vi "Script Controls (XML).vi"(11 "IDM Descriptor Array In":T1) -> (0 "error out":errorcluster, 1 "Terms to Show":string[](array[string]), 2 "Generated XML":string, 3 "IDM Descriptor Array Out":T1, 4 "Required Terms":i32[](array[numeric]))   [LabVIEW 2021]
uses:
  <vilib>/myRIO/Common/Express VI Framework/typedefs/Instrument Driver Method Descriptor Array.ctl
  <vilib>/myRIO/Common/Express VI Framework/typedefs/Instrument Driver Method Descriptor.ctl
  <vilib>/myRIO/Common/Express VI Framework/typedefs/Create FP Controls Actions.ctl
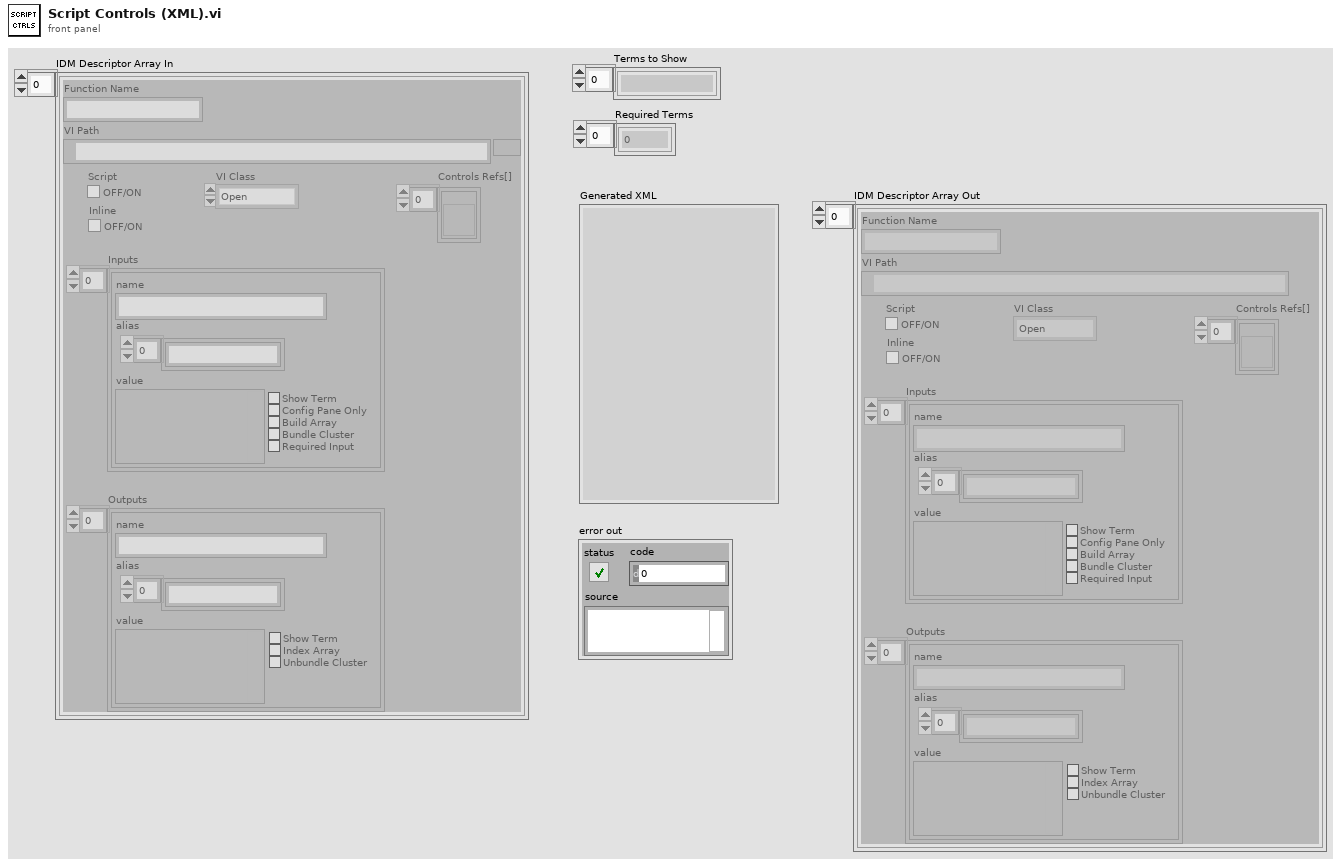
[diagram p1: front panel]
types:
  T1 = typedef "Instrument Driver Method Descriptor Array.ctl" = T2[]
  T2 = typedef "Instrument Driver Method Descriptor.ctl" = cluster{"Function Name":string, "VI Path":path, "Script":bool, "Inputs":cluster{"name":string, "value":variant, "Config Pane Only":bool, "Build Array":bool, "Bundle Cluster":bool, "Show Term":bool, "alias":string[], "Required Input":bool}[], "Outputs":cluster{"name":string, "value":variant, "Show Term":bool, "Index Array":bool, "Unbundle Cluster":bool, "alias":string[]}[], "VI Class":enum16{"Open", "Configure", "Data", "Manage", "Close"}, "Controls Refs[]":refnum<vi>[], "Inline":bool}
  T3 = typedef "Create FP Controls Actions.ctl" = enum16{"Create Control", "Create Indicator", "Create Constant", "Build Array", "Index Array", "Create Error In", "Create Error Out", "Bundle Cluster", "Unbundle Cluster"}
  T4 = cluster{"name":string, "value":variant, "Config Pane Only":bool, "Build Array":bool, "Bundle Cluster":bool, "Show Term":bool, "alias":string[], "Required Input":bool}[]
  T5 = cluster{"name":string, "value":variant, "Show Term":bool, "Index Array":bool, "Unbundle Cluster":bool, "alias":string[]}[]
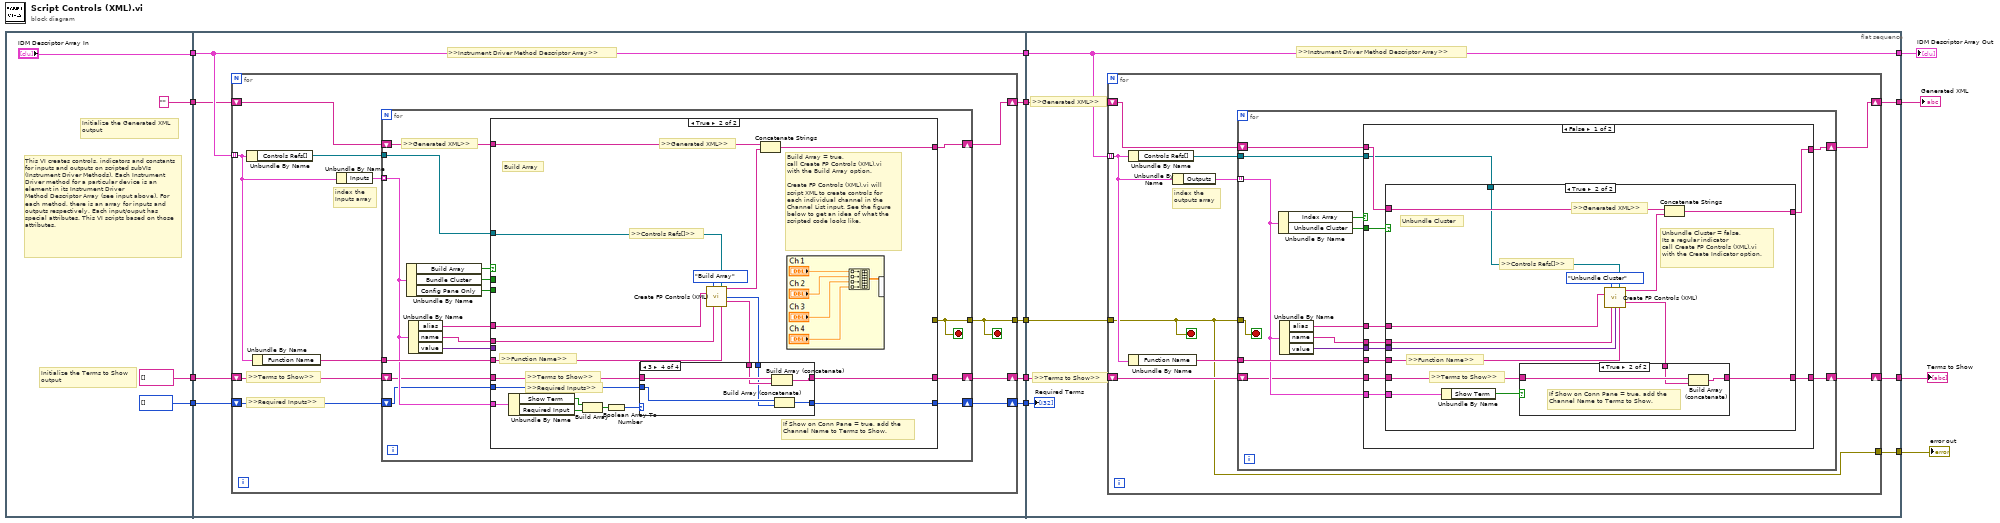
[diagram p0: block diagram]
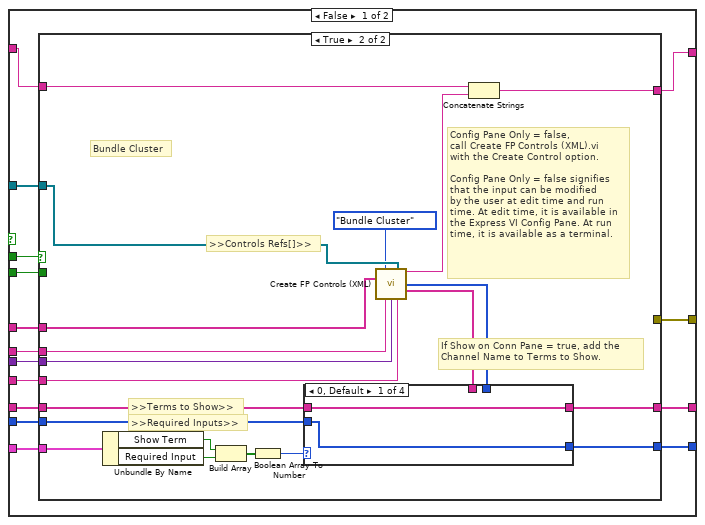
[diagram p2: hidden frame]
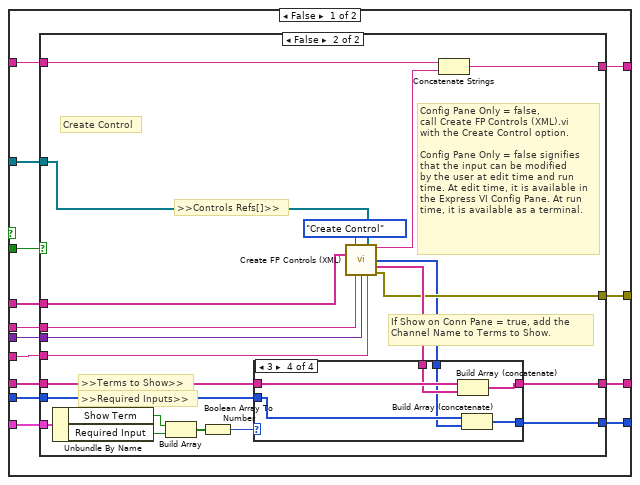
[diagram p3: hidden frame]
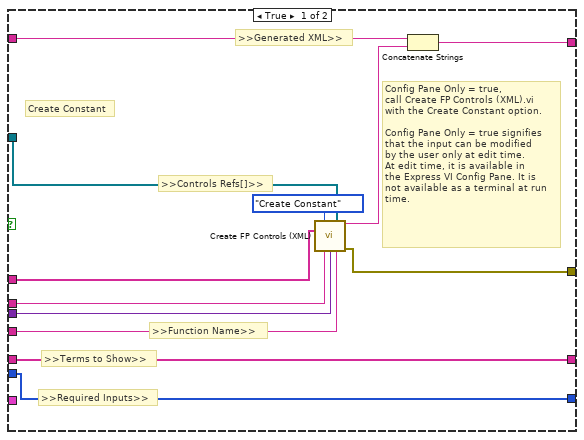
[diagram p4: hidden frame]
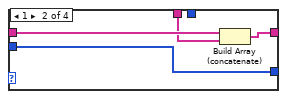
[diagram p6: hidden frame]
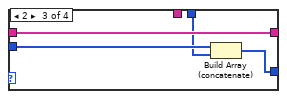
[diagram p7: hidden frame]
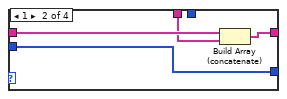
[diagram p8: hidden frame]
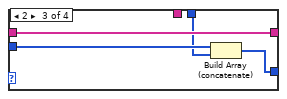
[diagram p9: hidden frame]
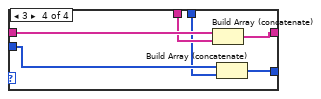
[diagram p10: hidden frame]
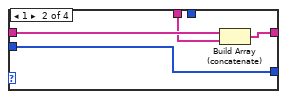
[diagram p12: hidden frame]
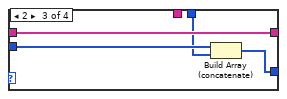
[diagram p13: hidden frame]
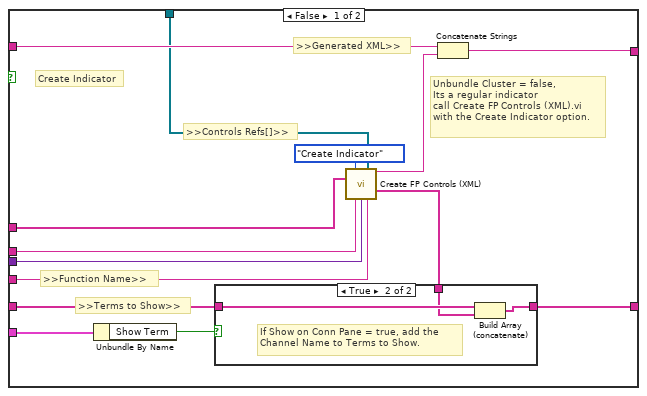
[diagram p14: hidden frame]
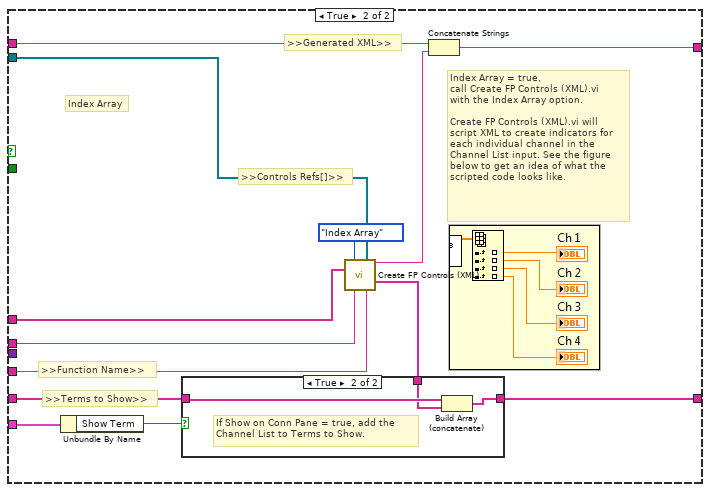
[diagram p17: hidden frame]
diagram:
  n1 = flat-sequence {
    tunnel: ["IDM Descriptor Array In"] -> w13
    tunnel: ["" ("Generated XML")] -> w11
    tunnel: [string[] [] ("array")] -> w8
    tunnel: [i32[] [] ("Required Terms")] -> w2
    tunnel: w13 -> [w25]
    tunnel: [w25] -> w12
    tunnel: w11 -> [w24]
    tunnel: [w23] -> w10
    tunnel: w8 -> [w22]
    tunnel: [w21] -> w7
    tunnel: [w20] -> w4
    tunnel: w2 -> [w19]
    tunnel: [w18] -> w1
    tunnel: w12 -> [w205]
    tunnel: w10 -> [w209]
    tunnel: [w208] -> w9
    tunnel: w7 -> [w207]
    tunnel: [w206] -> w6
    tunnel: [w205] -> w5
    tunnel: w4 -> [w204]
    tunnel: [w203] -> w3
    tunnel: w1 -> [w202]
    frame #0 {
      # "This VI creates controls, indicators and constants for inputs and outputs on scripted subVIs (Instrument Driver Methods). Each Instrument Driver method for a particular device is an element in its Instrument Driver \nMethod Descriptor Array (see input above). For each method, there is an array for inputs and outputs respectively. Each input/ouput has special attributes. This VI scripts based on those attributes."
      # "Initialize the Terms to Show\noutput"
      # "Initialize the Generated XML\noutput"
    }
    frame #1 {
      # ">>Instrument Driver Method Descriptor Array>>"
      n2 = for {
        tunnel: w25 -> [w36] mode=indexing
        shift-right: [w33] -> w23
        shift-left: w24 -> [w34]
        shift-right: [w31] -> w21
        shift-left: w22 -> [w32]
        tunnel: [w28] -> w20
        shift-right: [w26] -> w18
        shift-left: w19 -> [w27]
        stop <- w28 stop-if-true
        # ">>Required Inputs>>"
        # "index the \nInputs array"
        # ">>Terms to Show>>"
        n3 = Unbundle By Name(w36) -> ("Controls Refs[]"=w30:refnum<vi>[])
        n4 = Unbundle By Name(w36) -> ("Function Name"=w35:string)
        n5 = Unbundle By Name(w36) -> ("Inputs"=w29:T4)
        n6 = for {
          tunnel: w29 -> [w48] mode=indexing
          tunnel: w35 -> [w50]
          shift-right: [w44] -> w33
          shift-left: w34 -> [w45]
          tunnel: w30 -> [w43]
          shift-right: [w41] -> w31
          shift-left: w32 -> [w42]
          tunnel: [w39] -> w28
          shift-right: [w37] -> w26
          shift-left: w27 -> [w38]
          stop <- w39 stop-if-true
          # ">>Generated XML>>"
          n7 = Unbundle By Name(w48) -> ("Build Array"=w47:bool, "Bundle Cluster"=w46:bool, "Config Pane Only"=w52:bool)
          n8 = Unbundle By Name(w48) -> ("alias"=w40:string[], "name"=w51:string, "value"=w49:variant)
          n9 = case shown="True" w47 {
            tunnel: w52 -> [w67 _]
            tunnel: w51 -> [w66 w184]
            tunnel: w50 -> [w65 w183]
            tunnel: w49 -> [w64 _]
            tunnel: w48 -> [w63 w174]
            tunnel: w46 -> [w62 _]
            tunnel: w45 -> [w61 w181]
            tunnel: [w60 w182] -> w44
            tunnel: w43 -> [w59 w180]
            tunnel: w42 -> [w58 w176]
            tunnel: [w57 w171] -> w41
            tunnel: w40 -> [w56 w178]
            tunnel: [w55 _] -> w39
            tunnel: w38 -> [w54 w175]
            tunnel: [w53 w170] -> w37
            frame False {
              n10 = case shown="True" w62 {
                tunnel: w67 -> [w81 _]
                tunnel: w66 -> [w80 w150]
                tunnel: w65 -> [w79 w149]
                tunnel: w64 -> [w78 w148]
                tunnel: w63 -> [w77 w137]
                tunnel: w61 -> [w76 w147]
                tunnel: [w75 w146] -> w60
                tunnel: w59 -> [w74 w145]
                tunnel: w58 -> [w73 w139]
                tunnel: [w72 w134] -> w57
                tunnel: w56 -> [w71 w144]
                tunnel: [w70 _] -> w55
                tunnel: w54 -> [w69 w138]
                tunnel: [w68 w133] -> w53
                frame False {
                  n11 = case shown="False" w81 {
                    tunnel: w80 -> [w92 w113]
                    tunnel: w79 -> [w91 w112]
                    tunnel: w78 -> [w90 w111]
                    tunnel: w77 -> [_ w110]
                    tunnel: w76 -> [w89 w109]
                    tunnel: [w88 w108] -> w75
                    tunnel: w74 -> [w87 w107]
                    tunnel: w73 -> [w86 w106]
                    tunnel: [w86 w105] -> w72
                    tunnel: w71 -> [w84 w103]
                    tunnel: [w83 w101] -> w70
                    tunnel: w69 -> [w82 w96]
                    tunnel: [w82 w95] -> w68
                    frame True {
                      # ">>Required Inputs>>"
                      # ">>Generated XML>>"
                      # ">>Function Name>>"
                      # ">>Controls Refs[]>>"
                      # ">>Terms to Show>>"
                      # "Config Pane Only = true,\ncall Create FP Controls (XML).vi\nwith the Create Constant option.\n\nConfig Pane Only = true signifies\nthat the input can be modified\nby the user only at edit time. \nAt edit time, it is available in\nthe Express VI Config Pane. It is\nnot available as a terminal at run\ntime."
                      # "Create Constant"
                      n12 = call <vilib>:"Create FP Controls (XML).vi"("Action"=Create_FP_Controls_Actions."Create Constant", "Controls Refs[]"=w87, "Alias List"=w84, "Terminal Name"=w92, "Value"=w90, "Function Name"=w91) -> ("Generated XML"=w93:string, "error out"=w83:errorcluster)  [unwired: 6 in, 2 out]
                      n13 = Concatenate Strings(w89, w93) -> (w88:string)
                    }
                    frame False {
                      # ">>Required Inputs>>"
                      # "If Show on Conn Pane = true, add the \nChannel Name to Terms to Show."
                      # ">>Controls Refs[]>>"
                      # ">>Terms to Show>>"
                      # "Config Pane Only = false,\ncall Create FP Controls (XML).vi\nwith the Create Control option.\n\nConfig Pane Only = false signifies\nthat the input can be modified\nby the user at edit time and run \ntime. At edit time, it is available in\nthe Express VI Config Pane. At run\ntime, it is available as a terminal."
                      # "Create Control"
                      n14 = Unbundle By Name(w110) -> ("Show Term"=w100:bool, "Required Input"=w99:bool)
                      n15 = Build Array(w100, w99) -> (w98:bool[])
                      n16 = Boolean Array To Number(Boolean array=w98) -> (number=w97:u32)
                      n17 = call <vilib>:"Create FP Controls (XML).vi"("Action"=Create_FP_Controls_Actions."Create Control", "Controls Refs[]"=w107, "Alias List"=w103, "Terminal Name"=w113, "Value"=w111, "Function Name"=w112) -> ("Generated XML"=w114:string, "Input Terms"=w94:i32[], "Terms to Show"=w102:string[], "error out"=w101:errorcluster)  [unwired: 6 in]
                      n18 = case shown="3" w97 {
                        tunnel: w106 -> [w116 w120 w124 w130]
                        tunnel: [w116 w119 w124 w128] -> w105
                        tunnel: w102 -> [_ w118 _ w129]
                        tunnel: w96 -> [w115 w117 w123 w127]
                        tunnel: [w115 w117 w121 w125] -> w95
                        tunnel: w94 -> [_ _ w122 w126]
                        frame 0, Default {
                        }
                        frame 1 {
                          n19 = Build Array (concatenate)(w120, w118) -> (w119:string[])
                        }
                        frame 2 {
                          n20 = Build Array (concatenate)(w123, w122) -> (w121:i32[])
                        }
                        frame 3 {
                          n21 = Build Array (concatenate)(w130, w129) -> (w128:string[])
                          n22 = Build Array (concatenate)(w127, w126) -> (w125:i32[])
                        }
                      }
                      n23 = Concatenate Strings(w109, w114) -> (w108:string)
                    }
                  }
                }
                frame True {
                  # ">>Required Inputs>>"
                  # "If Show on Conn Pane = true, add the \nChannel Name to Terms to Show."
                  # ">>Terms to Show>>"
                  # ">>Controls Refs[]>>"
                  # "Config Pane Only = false,\ncall Create FP Controls (XML).vi\nwith the Create Control option.\n\nConfig Pane Only = false signifies\nthat the input can be modified\nby the user at edit time and run \ntime. At edit time, it is available in\nthe Express VI Config Pane. At run\ntime, it is available as a terminal."
                  # "Bundle Cluster"
                  n24 = Unbundle By Name(w137) -> ("Show Term"=w131:bool, "Required Input"=w132:bool)
                  n25 = Build Array(w131, w132) -> (w141:bool[])
                  n26 = Boolean Array To Number(Boolean array=w141) -> (number=w140:u32)
                  n27 = call <vilib>:"Create FP Controls (XML).vi"("Action"=Create_FP_Controls_Actions."Bundle Cluster", "Controls Refs[]"=w145, "Alias List"=w144, "Terminal Name"=w150, "Value"=w148, "Function Name"=w149) -> ("Generated XML"=w143:string, "Input Terms"=w136:i32[], "Terms to Show"=w135:string[])  [unwired: 6 in, 1 out]
                  n28 = case shown="0, Default" w140 {
                    tunnel: w139 -> [w152 w156 w160 w166]
                    tunnel: [w152 w155 w160 w164] -> w134
                    tunnel: w135 -> [_ w154 _ w165]
                    tunnel: w138 -> [w151 w153 w159 w163]
                    tunnel: [w151 w153 w157 w161] -> w133
                    tunnel: w136 -> [_ _ w158 w162]
                    frame 0, Default {
                    }
                    frame 1 {
                      n29 = Build Array (concatenate)(w156, w154) -> (w155:string[])
                    }
                    frame 2 {
                      n30 = Build Array (concatenate)(w159, w158) -> (w157:i32[])
                    }
                    frame 3 {
                      n31 = Build Array (concatenate)(w166, w165) -> (w164:string[])
                      n32 = Build Array (concatenate)(w163, w162) -> (w161:i32[])
                    }
                  }
                  n33 = Concatenate Strings(w147, w143) -> (w146:string)
                }
              }
            }
            frame True {
              # ">>Required Inputs>>"
              # "If Show on Conn Pane = true, add the \nChannel Name to Terms to Show."
              # ">>Terms to Show>>"
              # ">>Generated XML>>"
              # ">>Function Name>>"
              # ">>Controls Refs[]>>"
              # "Build Array"
              # "Build Array = true,\ncall Create FP Controls (XML).vi\nwith the Build Array option.\n\nCreate FP Controls (XML).vi will\nscript XML to create controls for\neach individual channel in the \nChannel List input. See the figure\nbelow to get an idea of what the \nscripted code looks like."
              n34 = Unbundle By Name(w174) -> ("Show Term"=w168:bool, "Required Input"=w167:bool)
              n35 = Build Array(w168, w167) -> (w169:bool[])
              n36 = Boolean Array To Number(Boolean array=w169) -> (number=w177:u32)
              n37 = call <vilib>:"Create FP Controls (XML).vi"("Action"=Create_FP_Controls_Actions."Build Array", "Controls Refs[]"=w180, "Alias List"=w178, "Terminal Name"=w184, "Function Name"=w183) -> ("Generated XML"=w185:string, "Input Terms"=w173:i32[], "Terms to Show"=w172:string[])  [unwired: 7 in, 1 out]
              n38 = case shown="3" w177 {
                tunnel: w176 -> [w187 w191 w195 w201]
                tunnel: [w187 w190 w195 w199] -> w171
                tunnel: w172 -> [_ w189 _ w200]
                tunnel: w175 -> [w186 w188 w194 w198]
                tunnel: [w186 w188 w192 w196] -> w170
                tunnel: w173 -> [_ _ w193 w197]
                frame 0, Default {
                }
                frame 1 {
                  n39 = Build Array (concatenate)(w191, w189) -> (w190:string[])
                }
                frame 2 {
                  n40 = Build Array (concatenate)(w194, w193) -> (w192:i32[])
                }
                frame 3 {
                  n41 = Build Array (concatenate)(w201, w200) -> (w199:string[])
                  n42 = Build Array (concatenate)(w198, w197) -> (w196:i32[])
                }
              }
              n43 = Concatenate Strings(w181, w185) -> (w182:string)
            }
          }
        }
      }
    }
    frame #2 {
      # ">>Instrument Driver Method Descriptor Array>>"
      # ">>Generated XML>>"
      # ">>Terms to Show>>"
      n44 = for {
        tunnel: w205 -> [w218] mode=indexing
        shift-right: [w215] -> w208
        shift-left: w209 -> [w216]
        shift-right: [w213] -> w206
        shift-left: w207 -> [w214]
        tunnel: w204 -> [w210]
        tunnel: [w210] -> w203
        stop <- w210 stop-if-true
        # "index the \noutputs array"
        n45 = Unbundle By Name(w218) -> ("Controls Refs[]"=w212:refnum<vi>[])
        n46 = Unbundle By Name(w218) -> ("Function Name"=w217:string)
        n47 = Unbundle By Name(w218) -> ("Outputs"=w211:T5)
        n48 = for {
          tunnel: w211 -> [w228] mode=indexing
          tunnel: w217 -> [w230]
          tunnel: w212 -> [w225]
          shift-right: [w223] -> w215
          shift-left: w216 -> [w224]
          shift-right: [w221] -> w213
          shift-left: w214 -> [w222]
          tunnel: w210 -> [w219]
          stop <- w219 stop-if-true
          n49 = Unbundle By Name(w228) -> ("Index Array"=w227:bool, "Unbundle Cluster"=w226:bool)
          n50 = Unbundle By Name(w228) -> ("alias"=w220:string[], "name"=w231:string, "value"=w229:variant)
          n51 = case shown="False" w227 {
            tunnel: w231 -> [w242 w290]
            tunnel: w230 -> [w241 w289]
            tunnel: w229 -> [w240 _]
            tunnel: w228 -> [w239 w287]
            tunnel: w226 -> [w238 _]
            tunnel: w225 -> [w235 w284]
            tunnel: w224 -> [w237 w286]
            tunnel: [w236 w285] -> w223
            tunnel: w222 -> [w234 w283]
            tunnel: [w233 w282] -> w221
            tunnel: w220 -> [w232 w280]
            frame False {
              n52 = case shown="True" w238 {
                tunnel: w242 -> [w256 w274]
                tunnel: w241 -> [w255 w273]
                tunnel: w240 -> [w254 w272]
                tunnel: w239 -> [w253 w271]
                tunnel: w237 -> [w250 w268]
                tunnel: [w249 w267] -> w236
                tunnel: w235 -> [w248 w266]
                tunnel: w234 -> [w247 w265]
                tunnel: [w246 w264] -> w233
                tunnel: w232 -> [w244 w262]
                frame False {
                  # ">>Terms to Show>>"
                  # ">>Function Name>>"
                  # ">>Controls Refs[]>>"
                  # ">>Generated XML>>"
                  # "Unbundle Cluster = false,\nIts a regular indicator\ncall Create FP Controls (XML).vi\nwith the Create Indicator option."
                  # "Create Indicator"
                  n53 = Unbundle By Name(w253) -> ("Show Term"=w251:bool)
                  n54 = call <vilib>:"Create FP Controls (XML).vi"("Action"=Create_FP_Controls_Actions."Create Indicator", "Controls Refs[]"=w248, "Alias List"=w244, "Terminal Name"=w256, "Value"=w254, "Function Name"=w255) -> ("Generated XML"=w252:string, "Terms to Show"=w243:string[])  [unwired: 6 in, 2 out]
                  n55 = case shown="True" w251 {
                    tunnel: w247 -> [w257 w260]
                    tunnel: [w257 w259] -> w246
                    tunnel: w243 -> [_ w258]
                    frame False {
                    }
                    frame True {
                      # "If Show on Conn Pane = true, add the \nChannel Name to Terms to Show."
                      n56 = Build Array (concatenate)(w260, w258) -> (w259:string[])
                    }
                  }
                  n57 = Concatenate Strings(w250, w252) -> (w249:string)
                }
                frame True {
                  # "Unbundle Cluster"
                  # ">>Terms to Show>>"
                  # ">>Function Name>>"
                  # ">>Controls Refs[]>>"
                  # ">>Generated XML>>"
                  # "Unbundle Cluster = false,\nIts a regular indicator\ncall Create FP Controls (XML).vi\nwith the Create Indicator option."
                  n58 = Unbundle By Name(w271) -> ("Show Term"=w269:bool)
                  n59 = call <vilib>:"Create FP Controls (XML).vi"("Action"=Create_FP_Controls_Actions."Unbundle Cluster", "Controls Refs[]"=w266, "Alias List"=w262, "Terminal Name"=w274, "Value"=w272, "Function Name"=w273) -> ("Generated XML"=w270:string, "Terms to Show"=w261:string[])  [unwired: 6 in, 2 out]
                  n60 = case shown="True" w269 {
                    tunnel: w265 -> [w275 w278]
                    tunnel: [w275 w277] -> w264
                    tunnel: w261 -> [_ w276]
                    frame False {
                    }
                    frame True {
                      # "If Show on Conn Pane = true, add the \nChannel Name to Terms to Show."
                      n61 = Build Array (concatenate)(w278, w276) -> (w277:string[])
                    }
                  }
                  n62 = Concatenate Strings(w268, w270) -> (w267:string)
                }
              }
            }
            frame True {
              # ">>Generated XML>>"
              # ">>Function Name>>"
              # ">>Controls Refs[]>>"
              # ">>Terms to Show>>"
              # "Index Array = true,\ncall Create FP Controls (XML).vi\nwith the Index Array option.\n\nCreate FP Controls (XML).vi will\nscript XML to create indicators for\neach individual channel in the \nChannel List input. See the figure\nbelow to get an idea of what the \nscripted code looks like."
              # "Index Array"
              n63 = Unbundle By Name(w287) -> ("Show Term"=w288:bool)
              n64 = call <vilib>:"Create FP Controls (XML).vi"("Action"=Create_FP_Controls_Actions."Index Array", "Controls Refs[]"=w284, "Alias List"=w280, "Terminal Name"=w290, "Function Name"=w289) -> ("Generated XML"=w291:string, "Terms to Show"=w279:string[])  [unwired: 7 in, 2 out]
              n65 = case shown="True" w288 {
                tunnel: w283 -> [w292 w295]
                tunnel: [w292 w294] -> w282
                tunnel: w279 -> [_ w293]
                frame False {
                }
                frame True {
                  # "If Show on Conn Pane = true, add the \nChannel List to Terms to Show."
                  n66 = Build Array (concatenate)(w295, w293) -> (w294:string[])
                }
              }
              n67 = Concatenate Strings(w286, w291) -> (w285:string)
            }
          }
        }
      }
      "Required Terms" <- w202
    }
  }
  "Generated XML" <- w9
  "Terms to Show" <- w6
  "IDM Descriptor Array Out" <- w5
  "error out" <- w3
